vi "AcqStatus.vi"(6 "FramesToCollect":u32, 7 "Acq Params":T1, 9 "Galvo Record":T2, 10 "Digital Signals":cluster{"StartTrig":bool, "LaserClk":bool}, 11 "data in":T5={"channel 0"=[0, 0], "channel 1"=[0, 0], "channel 2"=[0, 0], "channel 3"=[0, 0], "channel 4"=[0, 0], "channel 5"=[0, 0], "channel 6"=[0, 0], "channel 7"=[0, 0]}) -> (0 "AcqStatus":T4, 1 "AcqSatus":T3, 2 "GalvoSamplesRemaining":u32, 3 "data out":T5, 4 "FramesDone":u32)   [LabVIEW 2015]
uses:
  Typedefs/AcqStatus.ctl
  Typedefs/StateMachineStates.ctl
  <vilib>/rvi/eio/common/nirviEmuTemplateMethod_errors.vi
  <vilib>/eio/EIOMethodNode/EIOMethodNode.xnode
  <vilib>/eio/EIONode/EIONode.xnode
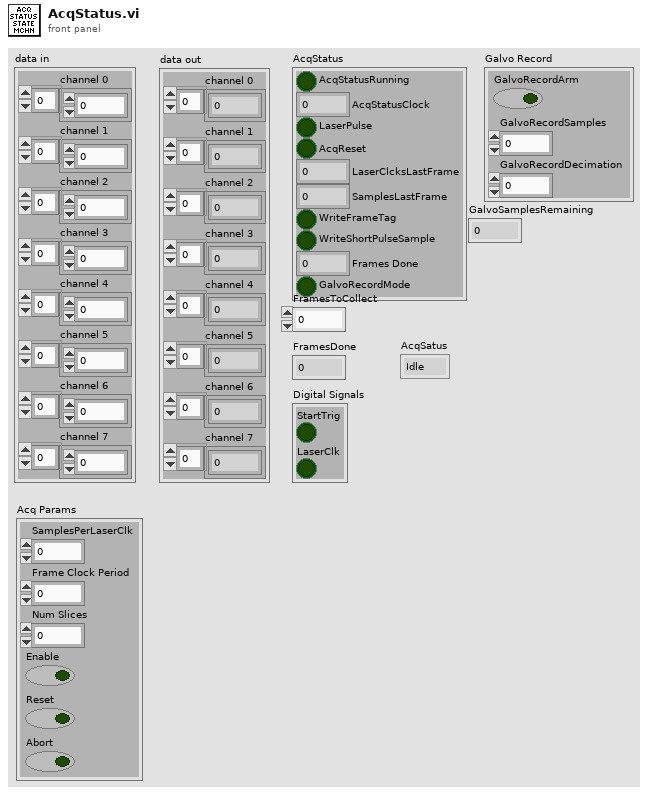
[diagram p1: front panel]
types:
  T1 = cluster{"SamplesPerLaserClk":u8, "Frame Clock Period":u64, "Num Slices":u16, "Enable":bool, "Reset":bool, "Abort":bool}
  T2 = cluster{"GalvoRecordArm":bool, "GalvoRecordSamples":u32, "GalvoRecordDecimation":u32}
  T3 = typedef "StateMachineStates.ctl" = enum16{"Idle", "Armed", "Running", "Galvo Record Armed", "Galvo Recording"}
  T4 = typedef "AcqStatus.ctl" = cluster{"AcqStatusRunning":bool, "AcqStatusClock":u64, "LaserPulse":bool, "AcqReset":bool, "LaserClcksLastFrame":u32, "SamplesLastFrame":u32, "WriteFrameTag":bool, "WriteShortPulseSample":bool, "Frames Done":u32, "GalvoRecordMode":bool}
  T5 = cluster{"channel 0":i16[], "channel 1":i16[], "channel 2":i16[], "channel 3":i16[], "channel 4":i16[], "channel 5":i16[], "channel 6":i16[], "channel 7":i16[]}
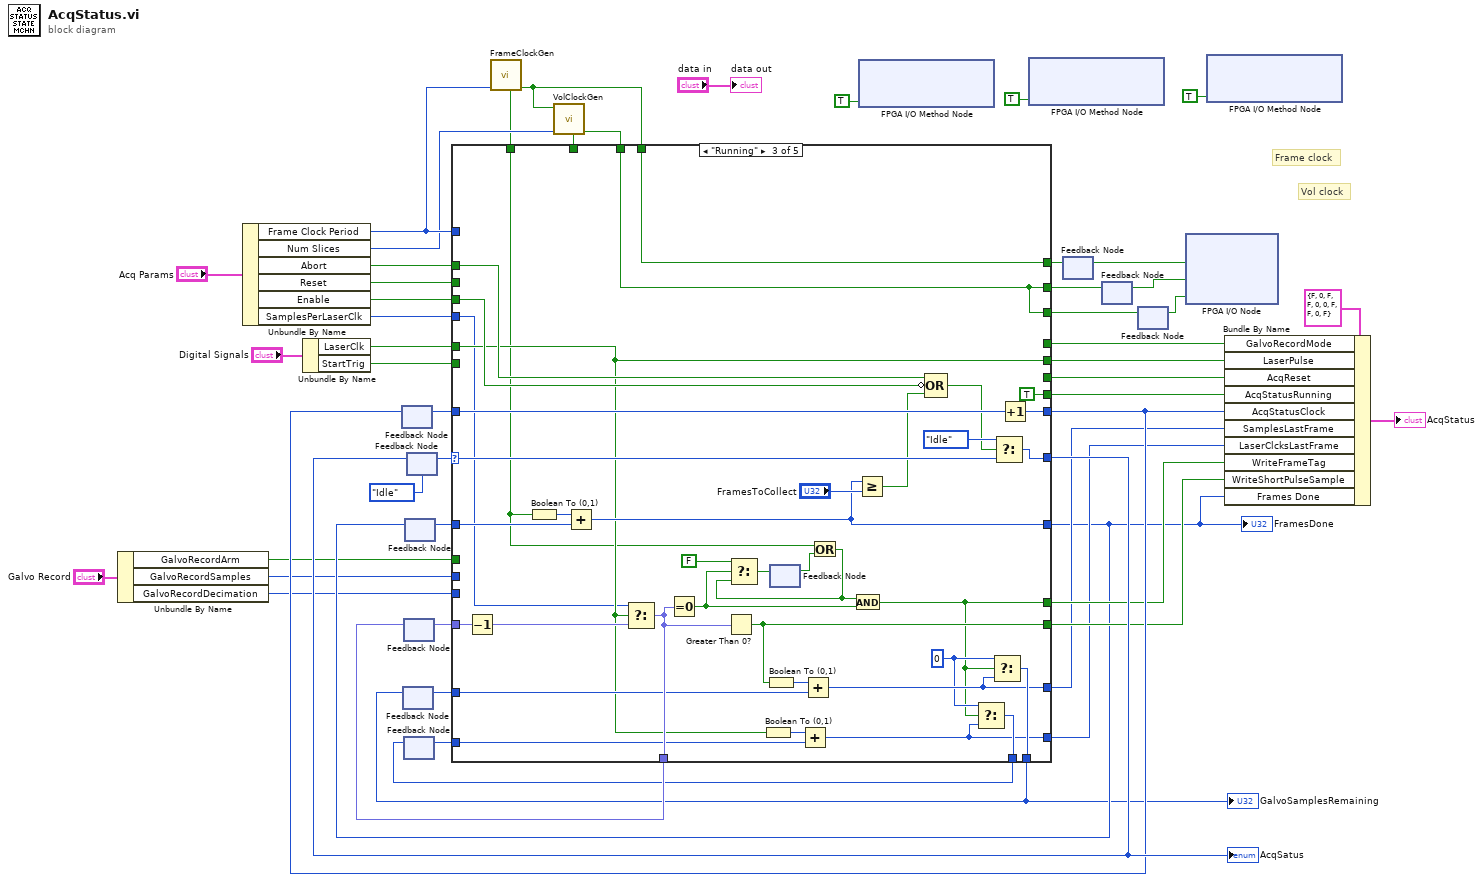
[diagram p0: block diagram]
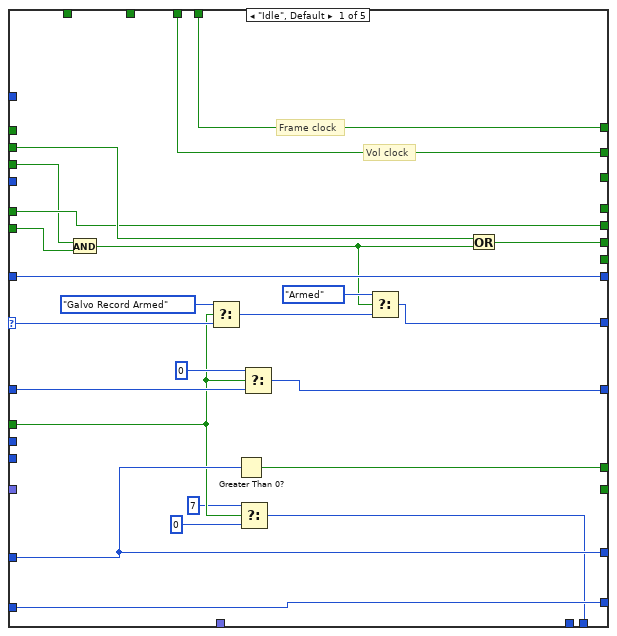
[diagram p2: hidden frame]
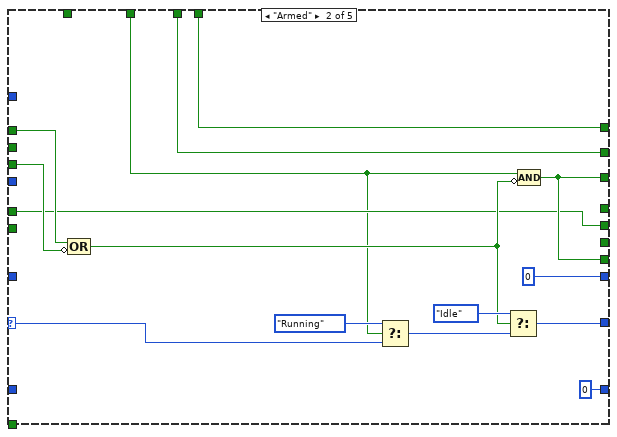
[diagram p3: hidden frame]
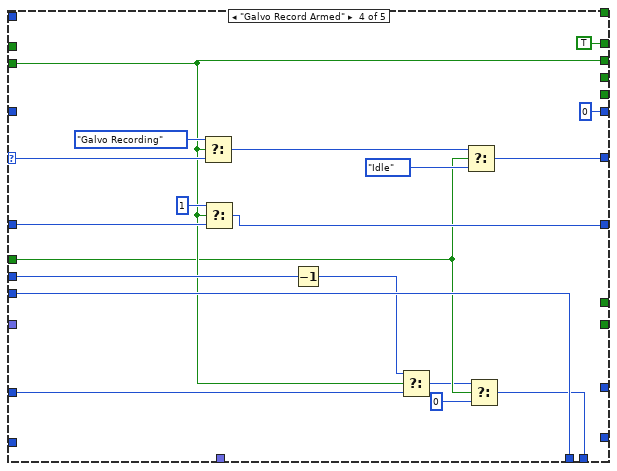
[diagram p4: hidden frame]
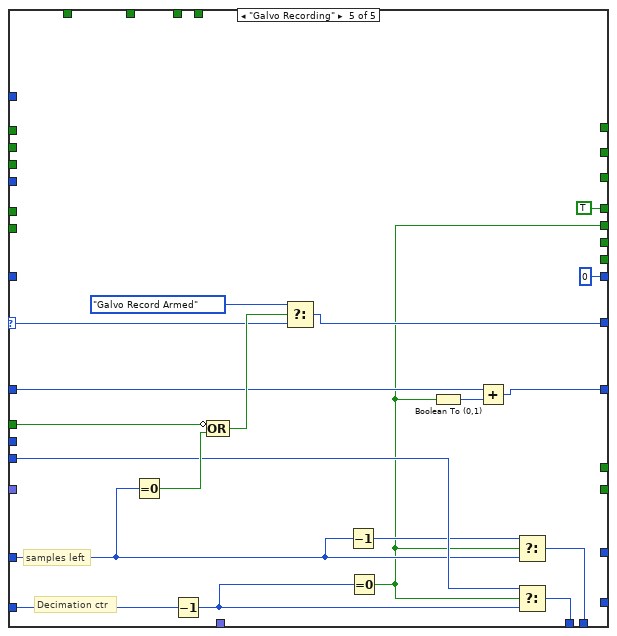
[diagram p5: hidden frame]
diagram:
  # "Frame clock"
  # "Vol clock"
  n1 = Unbundle By Name("Galvo Record") -> ("GalvoRecordArm"=w25:bool, "GalvoRecordSamples"=w24:u32, "GalvoRecordDecimation"=w23:u32)
  n2 = Unbundle By Name("Acq Params") -> ("Frame Clock Period"=w9:u64, "Num Slices"=w8:u16, "Abort"=w16:bool, "Reset"=w15:bool, "Enable"=w14:bool, "SamplesPerLaserClk"=w13:u8)
  n3 = Unbundle By Name("Digital Signals") -> ("LaserClk"=w36:bool, "StartTrig"=w50:bool)
  n4 = feedback #1() -> (w43:u64)  [unwired: 1 in]
  n5 = feedback #2() -> (w39:u32)  [unwired: 1 in]
  n6 = feedback #3() -> (w37:fxp<+,8,8>)  [unwired: 1 in]
  n7 = feedback #4() -> (w38:u32)  [unwired: 1 in]
  n8 = feedback #5() -> (w41:u32)  [unwired: 1 in]
  n9 = feedback #6(StateMachineStates."Idle") -> (w48:T3)
  n10 = call "FrameClockGen.vi"("Clock Period"=w9) -> ("Pulse"=w6:bool, "Pulse Start"=w4:bool)  [unwired: 9 in]
  n11 = call "VolClockGen.vi"("Num Slices"=w8, "Frame Clk In"=w6) -> ("Volume Clk Out"=w7:bool, "Pulse Start"=w5:bool)  [unwired: 8 in]
  n12 = case shown="\"Running\"" w48 {
    selector: w48 -> [w66 w83 w124 w146 w163]
    tunnel: w50 -> [w54 _ _ w133 _]
    tunnel: w16 -> [_ w87 w121 _ _]
    tunnel: [w75 w86 w123 w142 w162] -> w46
    tunnel: w14 -> [w55 w88 w122 _ _]
    tunnel: [w67 _ _ _ _] -> w45
    tunnel: [_ w80 TRUE _ _] -> w44
    tunnel: [w73 u64 0 ("(hi.lo)") w126 u64 0 ("(hi.lo)") u64 0 ("(hi.lo)")] -> w42
    tunnel: w43 -> [w73 _ w127 _ _]
    tunnel: w41 -> [w63 _ w117 w138 w151]
    tunnel: [w61 u32 0 w115 w137 w150] -> w29
    tunnel: w39 -> [w70 _ w104 w134 w153]
    tunnel: [w70 _ w102 _ _] -> w30
    tunnel: [_ _ w105 _ _] -> w33
    tunnel: w38 -> [w72 _ w98 _ w159]
    tunnel: w37 -> [_ _ w114 _ _]
    tunnel: w36 -> [w56 w79 w95 _ _]
    tunnel: [w71 _ w96 _ _] -> w35
    tunnel: [_ _ w106 _ _] -> w34
    tunnel: [w59 _ w103 w129 w155] -> w20
    tunnel: [_ _ w100 w140 w158] -> w32
    tunnel: [w72 _ w97 _ _] -> w31
    tunnel: w15 -> [w68 _ _ _ _]
    tunnel: [_ w80 w91 _ _] -> w28
    tunnel: w25 -> [w60 _ _ w132 w165]
    tunnel: w24 -> [_ _ _ w141 _]
    tunnel: w23 -> [_ _ _ w140 w157]
    tunnel: [w56 w79 w95 w133 w148] -> w22
    tunnel: [_ _ _ TRUE TRUE] -> w21
    tunnel: [w52 w77 w91 _ _] -> w19
    tunnel: w9 -> [_ _ _ _ _]
    tunnel: w13 -> [_ _ w94 _ _]
    tunnel: [w53 w78 w92 _ _] -> w10
    tunnel: w6 -> [w53 w78 w92 _ _]
    tunnel: w7 -> [w52 w77 w91 _ _]
    tunnel: w5 -> [_ w76 _ _ _]
    tunnel: w4 -> [_ _ w93 _ _]
    frame "Idle", Default {
      # "Vol clock"
      # "Frame clock"
      n13 = And(x=w55, y=w54) -> (x .and. y?=w69:bool)
      n14 = Select(t=StateMachineStates."Galvo Record Armed", s=w60, f=w66) -> (s? t:f=w65:T3)
      n15 = Greater Than 0?(x=w70) -> (x > 0?=w71:bool)
      n16 = Select(t=u32 7, s=w60, f=u32 0 ("t")) -> (s? t:f=w59:u32)
      n17 = Select(t=u32 0, s=w60, f=w63) -> (s? t:f=w61:u32)
      n18 = Select(t=StateMachineStates."Armed", s=w69, f=w65) -> (s? t:f=w75:T3)
      n19 = Or(x=w68, y=w69) -> (x .or. y?=w67:bool)
    }
    frame "Armed" {
      n20 = Compound Arithmetic op=OR(w87, invert w88) -> (w82:bool)
      n21 = Select(t=StateMachineStates."Running", s=w76, f=w83) -> (s? t:f=w84:T3)
      n22 = Select(t=StateMachineStates."Idle", s=w82, f=w84) -> (s? t:f=w86:T3)
      n23 = Compound Arithmetic op=AND(w76, invert w82) -> (w80:bool)
    }
    frame "Running" {
      w101 = u32 0 ("t")
      n24 = Decrement(x=w114) -> (x-1=w113:fxp<+,8,8>)
      n25 = Boolean To (0,1)(Boolean=w93) -> (0, 1=w116:i16)
      n26 = Add(x=w116, y=w117) -> (x+y=w115:u32)
      n27 = Select(t=w94, s=w95, f=w113) -> (s? t:f=w106:fxp<+,8,8>)
      n28 = Equal To 0?(x=w106) -> (x = 0?=w109:bool)
      n29 = Greater Than 0?(x=w106) -> (x > 0?=w105:bool)
      n30 = Boolean To (0,1)(Boolean=w95) -> (0, 1=w99:i16)
      n31 = Boolean To (0,1)(Boolean=w105) -> (0, 1=w107:i16)
      n32 = feedback #7() -> (w111:bool)  [unwired: 1 in]
      n33 = Add(x=w99, y=w98) -> (x+y=w97:u32)
      n34 = Add(x=w107, y=w104) -> (x+y=w102:u32)
      n35 = Or(x=w93, y=w111) -> (x .or. y?=w108:bool)
      n36 = Select(t=FALSE, s=w109, f=w108) -> (s? t:f=w112:bool)
      n37 = feedback-in #7(w112) -> ()
      n38 = And(x=w108, y=w109) -> (x .and. y?=w96:bool)
      n39 = Greater Or Equal?(x=w115, y="FramesToCollect") -> (x >= y?=w118:bool)
      n40 = Compound Arithmetic op=OR(w121, invert w122, w118) -> (w120:bool)
      n41 = Select(t=w101, s=w96, f=w97) -> (s? t:f=w100:u32)
      n42 = Select(t=w101, s=w96, f=w102) -> (s? t:f=w103:u32)
      n43 = Select(t=StateMachineStates."Idle", s=w120, f=w124) -> (s? t:f=w123:T3)
      n44 = Increment(x=w127) -> (x+1=w126:u64)
    }
    frame "Galvo Record Armed" {
      n45 = Select(t=StateMachineStates."Galvo Recording", s=w133, f=w146) -> (s? t:f=w144:T3)
      n46 = Select(t=u32 1, s=w133, f=w138) -> (s? t:f=w137:u32)
      n47 = Decrement(x=w141) -> (x-1=w135:u32)
      n48 = Select(t=w135, s=w133, f=w134) -> (s? t:f=w130:u32)
      n49 = Select(t=w144, s=w132, f=StateMachineStates."Idle") -> (s? t:f=w142:T3)
      n50 = Select(t=w130, s=w132, f=u32 0 ("t")) -> (s? t:f=w129:u32)
    }
    frame "Galvo Recording" {
      # "samples left"
      # "Decimation ctr"
      n51 = Equal To 0?(x=w153) -> (x = 0?=w160:bool)
      n52 = Decrement(x=w159) -> (x-1=w156:u32)
      n53 = Compound Arithmetic op=OR(invert w165, w160) -> (w164:bool)
      n54 = Select(t=StateMachineStates."Galvo Record Armed", s=w164, f=w163) -> (s? t:f=w162:T3)
      n55 = Decrement(x=w153) -> (x-1=w154:u32)
      n56 = Equal To 0?(x=w156) -> (x = 0?=w148:bool)
      n57 = Boolean To (0,1)(Boolean=w148) -> (0, 1=w149:i16)
      n58 = Add(x=w151, y=w149) -> (x+y=w150:u32)
      n59 = Select(t=w154, s=w148, f=w153) -> (s? t:f=w155:u32)
      n60 = Select(t=w157, s=w148, f=w156) -> (s? t:f=w158:u32)
    }
  }
  "FramesDone" <- w29
  "AcqSatus" <- w46
  "GalvoSamplesRemaining" <- w20
  n61 = feedback-in #1(w42) -> ()
  n62 = feedback-in #2(w20) -> ()
  n63 = feedback-in #3(w34) -> ()
  n64 = feedback-in #4(w32) -> ()
  n65 = feedback-in #5(w29) -> ()
  n66 = feedback-in #6(w46) -> ()
  n67 = xnode "FPGA I/O Method Node"("Enable"=TRUE) -> ()  [unwired: 1 in, 1 out]
  n68 = xnode "FPGA I/O Method Node"("Enable"=TRUE) -> ()  [unwired: 1 in, 1 out]
  n69 = feedback-in #8(w10) -> ()
  n70 = feedback #8() -> (w1:bool)  [unwired: 1 in]
  n71 = feedback-in #9(w19) -> ()
  n72 = feedback #9() -> (w2:bool)  [unwired: 1 in]
  n73 = feedback-in #10(w28) -> ()
  n74 = feedback #10() -> (w3:bool)  [unwired: 1 in]
  n75 = xnode "FPGA I/O Node"("PXI_Trig4"=w1, "PXI_Trig5"=w2, "PXI_Trig6"=w3) -> ()  [unwired: 3 in, 3 out]
  n76 = xnode "FPGA I/O Method Node"("Enable"=TRUE) -> ()  [unwired: 1 in, 1 out]
  n77 = Bundle By Name(cluster=T4 {"AcqStatusRunning"=FALSE, "AcqStatusClock"=0, "LaserPulse"=FALSE, "AcqReset"=FALSE, "LaserClcksLastFrame"=0, "SamplesLastFrame"=0, "WriteFrameTag"=FALSE, "WriteShortPulseSample"=FALSE, "Frames Done"=0, "GalvoRecordMode"=FALSE} ("AcqStatus"), "GalvoRecordMode"=w21, "LaserPulse"=w22, "AcqReset"=w45, "AcqStatusRunning"=w44, "AcqStatusClock"=w42, "SamplesLastFrame"=w30, "LaserClcksLastFrame"=w31, "WriteFrameTag"=w35, "WriteShortPulseSample"=w33, "Frames Done"=w29) -> (→"AcqStatus":T4)
  "data out" <- "data in"
